vi "SIN.vi"() -> ()   [LabVIEW 2018]
uses:
  <vilib>/gmath/NI_Gmath.lvlib
panel:
  out "Waveform Chart":dbl(graph)
  out "sin(x)":dbl
  in  "x":dbl
  out "sin(x)":dbl
  in  "X":dbl
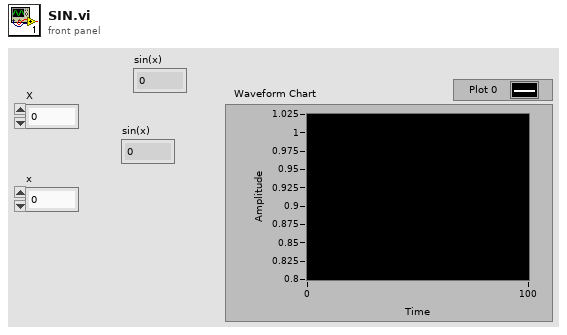
[diagram p1: front panel]
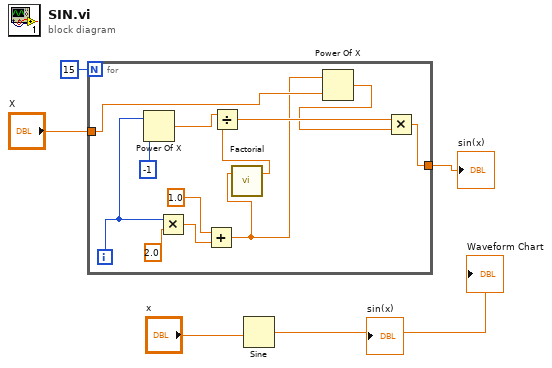
[diagram p0: block diagram]
diagram:
  n1 = for {
    N: 15 -> [_]
    tunnel: "X" -> [w12]
    tunnel: [w9] -> w3
    i -> [w8]
    n2 = Power Of X(1:-1 ("x"), 2:w8) -> (0:w13:dbl)
    n3 = Multiply(x=w8, y=2.0) -> (x*y=w15:dbl)
    n4 = Add(x=1.0 ("y"), y=w15) -> (x+y=w7:dbl)
    n5 = call <vilib>:"Factorial.vi"("n"=w7) -> ("n!"=w6:dbl)  [unwired: 2 in]
    n6 = Divide(x=w13, y=w6) -> (x/y=w11:dbl)
    n7 = Power Of X(1:w12, 2:w7) -> (0:w10:dbl)
    n8 = Multiply(x=w11, y=w10) -> (x*y=w9:dbl)
  }
  "sin(x)" <- w3
  n9 = Sine(x="x") -> (sin(x)=→"sin(x)" →"Waveform Chart":dbl)
